vi "test Counter-Driven Output.vi"(8 "error in (no error)":errorcluster, 11 "TestCase in":refnum<class "Scan Engine cRIO System Tests.lvclass">) -> (0 "error out":errorcluster, 3 "TestCase out":refnum<class "Scan Engine cRIO System Tests.lvclass">)   [LabVIEW 2016, in "Scan Engine cRIO System Tests.lvclass"]
uses:
  Scan Engine cRIO System Tests.lvclass
  C:/Users/rzoeller/Documents/ni-official/niveristand-custom-device-testing-tools/VeriStandTestCase/VeriStandTestCase.lvclass
  <vilib>/NI Veristand/Execution/Workspace/NI VeriStand - Get Single Channel Value.vi
  <vilib>/addons/_JKI Toolkits/VI Tester/TestCase.llb/TestCase.lvclass
  <vilib>/NI VeriStand/Execution/Workspace/NI_VS Workspace ExecutionAPI.lvlib
  C:/Program Files (x86)/National Instruments/LabVIEW 2016/vi.lib/addons/_JKI Toolkits/VI Tester/TestCase.llb/TestCase.lvclass
panel:
  in  "Terminal Count":i32=10
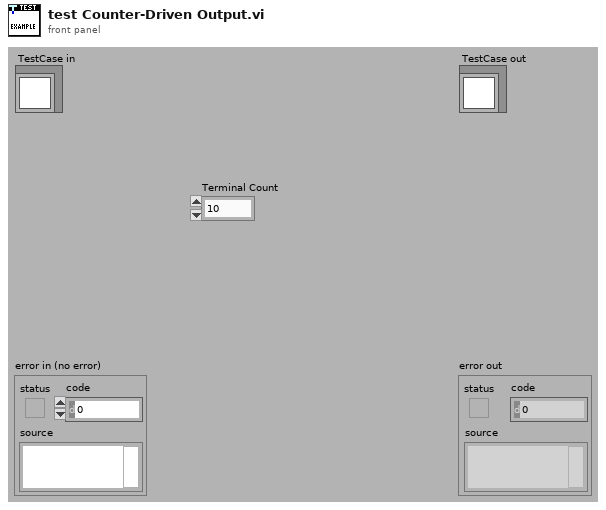
[diagram p1: front panel]
types:
  T1 = typedef "NI_VS Workspace ExecutionAPI.lvlib/WorkspaceAPI.ctl" = refnum<k24>
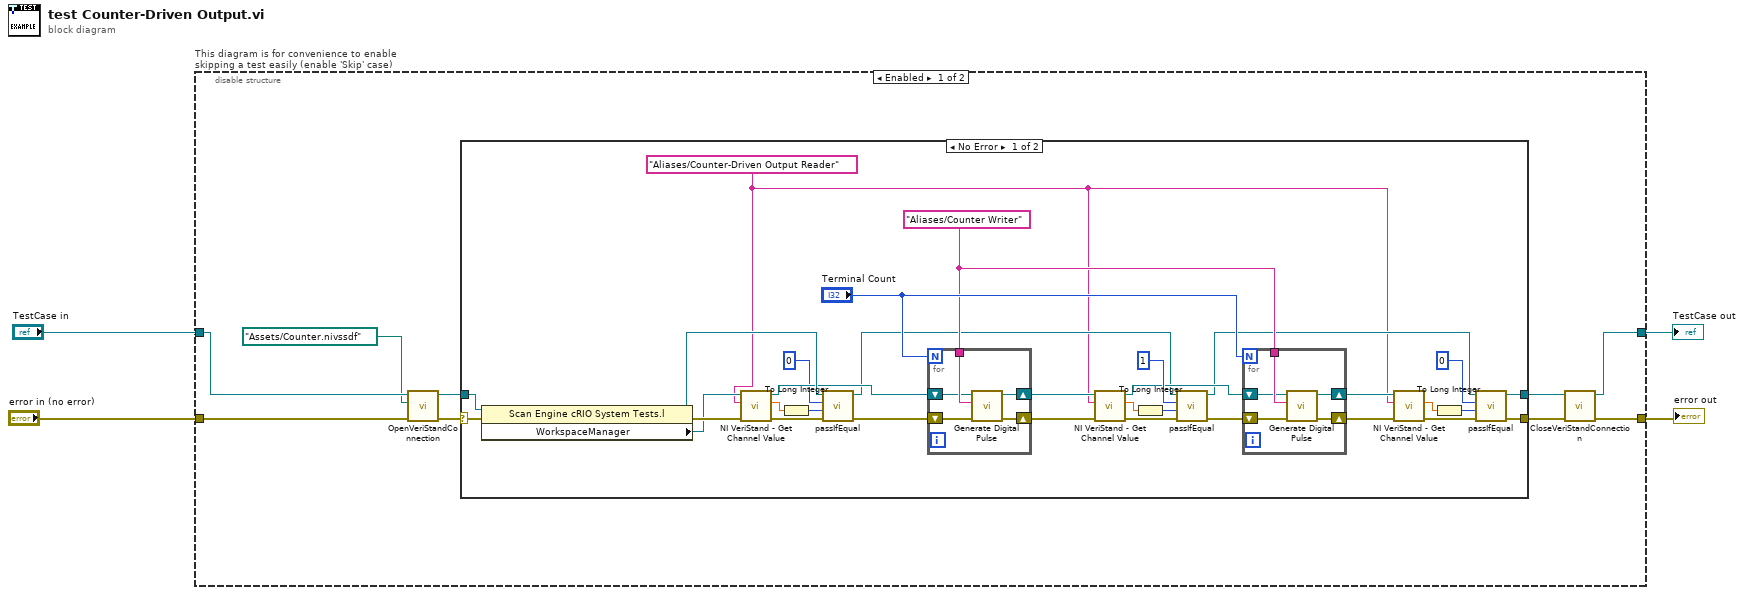
[diagram p0: block diagram]
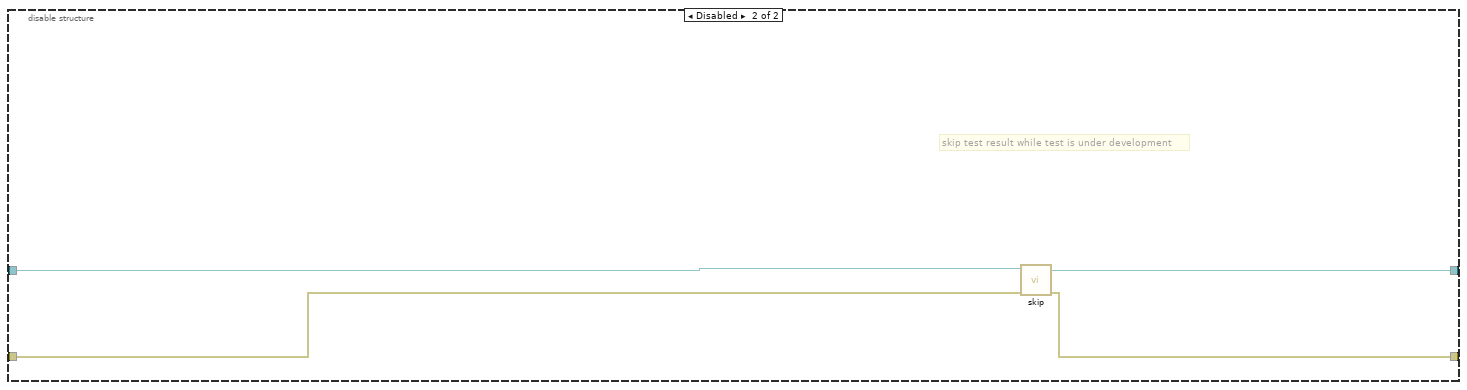
[diagram p3: hidden frame]
diagram:
  n1 = disable-structure "This diagram is for convenience to enable skipping a test easily (enable 'Skip' case)" shown="Enabled" {
    disable-tunnel: "TestCase in" -> [w13 w61]
    disable-tunnel: [w8 w59] -> w1
    disable-tunnel: [w6 w60] -> w3
    disable-tunnel: "error in (no error)" -> [w10 w58]
    frame Enabled {
      n2 = call-dynamic "OpenVeriStandConnection.vi"("error in (no error)"=w10, "System Definition File"=path "Assets/Counter.nivssdf", "VeriStand Test Case in"=w13) -> ("error out"=w11:errorcluster, "VeriStand Test Case out"=w12:refnum<class "Scan Engine cRIO System Tests.lvclass">)  [unwired: 7 in]
      n3 = case shown="No Error" w11 {
        selector: w11 -> [w16 w56]
        tunnel: w12 -> [w17 w57]
        tunnel: [w15 w57] -> w9
        tunnel: [w14 w56] -> w7
        frame No Error {
          w18 = "Aliases/Counter-Driven Output Reader" ("Channel")
          w35 = "Aliases/Counter Writer" ("Channel")
          n4 = property class="Scan Engine cRIO System Tests.l"(reference=w17, error in=w16) -> (reference out=w44:refnum<class "Scan Engine cRIO System Tests.lvclass">, error out=w43:errorcluster, "WorkspaceManager"=w41:T1)
          n5 = call-poly <vilib>:"NI VeriStand - Get Channel Value.vi"("error in (no error)"=w43, "Channel"=w18, "WorkspaceManager in"=w41) -> ("error out"=w42:errorcluster, "Value"=w39:dbl, "WorkspaceManager out"=w40:T1)  [unwired: 6 in]
          n6 = To Long Integer(number=w39) -> (32bit integer=w38:i32)
          n7 = call-dynamic "passIfEqual.vi"("error in (no error)"=w42, "y"=w38, "x"=0, "TestCase in"=w44) -> ("error out"=w45:errorcluster, "TestCase out"=w26:refnum<class "Scan Engine cRIO System Tests.lvclass">)  [unwired: 6 in]
          n8 = for {
            N: "Terminal Count" -> [_]
            shift-right: [w54] -> w29
            shift-left: w45 -> [w55]
            tunnel: w35 -> [w53]
            shift-right: [w51] -> w28
            shift-left: w40 -> [w52]
            n9 = call "Generate Digital Pulse.vi"("error in (no error)"=w55, "Channel"=w53, "WorkspaceManager"=w52) -> ("error out"=w54:errorcluster, "Workspace Manager out"=w51:T1)  [unwired: 7 in]
          }
          n10 = call-poly <vilib>:"NI VeriStand - Get Channel Value.vi"("error in (no error)"=w29, "Channel"=w18, "WorkspaceManager in"=w28) -> ("error out"=w34:errorcluster, "Value"=w33:dbl, "WorkspaceManager out"=w27:T1)  [unwired: 6 in]
          n11 = To Long Integer(number=w33) -> (32bit integer=w32:i32)
          n12 = call-dynamic "passIfEqual.vi"("error in (no error)"=w34, "y"=w32, "x"=1, "TestCase in"=w26) -> ("error out"=w30:errorcluster, "TestCase out"=w20:refnum<class "Scan Engine cRIO System Tests.lvclass">)  [unwired: 6 in]
          n13 = for {
            N: "Terminal Count" -> [_]
            shift-right: [w49] -> w21
            shift-left: w30 -> [w50]
            tunnel: w35 -> [w48]
            shift-right: [w46] -> w19
            shift-left: w27 -> [w47]
            n14 = call "Generate Digital Pulse.vi"("error in (no error)"=w50, "Channel"=w48, "WorkspaceManager"=w47) -> ("error out"=w49:errorcluster, "Workspace Manager out"=w46:T1)  [unwired: 7 in]
          }
          n15 = call-poly <vilib>:"NI VeriStand - Get Channel Value.vi"("error in (no error)"=w21, "Channel"=w18, "WorkspaceManager in"=w19) -> ("error out"=w25:errorcluster, "Value"=w24:dbl)  [unwired: 6 in, 1 out]
          n16 = To Long Integer(number=w24) -> (32bit integer=w23:i32)
          n17 = call-dynamic "passIfEqual.vi"("error in (no error)"=w25, "y"=w23, "x"=0, "TestCase in"=w20) -> ("error out"=w14:errorcluster, "TestCase out"=w15:refnum<class "Scan Engine cRIO System Tests.lvclass">)  [unwired: 6 in]
        }
        frame Error {
        }
      }
      n18 = call-dynamic "CloseVeriStandConnection.vi"("error in (no error)"=w7, "VeriStand Test Case in"=w9) -> ("error out"=w6:errorcluster, "VeriStand Test Case out"=w8:refnum<class "Scan Engine cRIO System Tests.lvclass">)  [unwired: 8 in]
    }
    frame Disabled {
      # "skip test result while test is under development"
      n19 = call <vilib>:"skip.vi"("error in (no error)"=w58, "TestCase in"=w61) -> ("error out"=w60:errorcluster, "TestCase out"=w59:refnum<class "Scan Engine cRIO System Tests.lvclass">)  [unwired: 8 in]
    }
  }
  "error out" <- w3
  "TestCase out" <- w1
